vi "G-Unicode Constant Editor.vi"(6 "Variant in":variant, 7 "Shift Pressed?":bool, 8 "error in (no error)":errorcluster, 10 "QD Combo Box Ref":refnum<vi>, 11 "QD Launch VI Ref":refnum<vi>) -> (0 "error out":errorcluster, 4 "Variant out":variant)   [LabVIEW 2020]
doc: "View and edit a constant UTF-8 string or UTF-8 path.\n\nDefault Shortcut - [G]"
uses:
  Types/UTF-8 String/UTF-8 String.lvclass
  Types/UTF-8 String/UTF-8 String.lvclass/UTF-8 String.ctl
  cd947f18-06e6-4942-b232-f387c9ba60e9.vi
  Private/Conversion/String as Encoded String.vi
  Private/Conversion/Polymorphic VIs/String as Encoded String (LabVIEW String).vi
  Private/Conversion/Polymorphic VIs/String as Encoded String (UTF-8 String).vi
  Types/UTF-8 String/Write Encoded UTF-8 String.vi
  Private/Conversion/Text to UTF-8.vi
  Private/Conversion/Polymorphic VIs/Text to UTF-8 (LabVIEW String).vi
  Types/UTF-8 String/Read Encoded UTF-8 String.vi
  Private/Library/gu_input_box.vi
  aec64f6a-b3cd-45af-92d8-e7d8603af3b4.vi
  Types/UTF-8 Path/UTF-8 Path.lvclass
  98fca13f-b951-49ec-b676-3ccf9bd4e781.vi
  5e95c1c1-3841-484b-b44d-c44c65ed04ae.vi
panel:
  in  "Undo Name":string="Quick Drop Keyboard Shortcut"
  # "Do not change the connector pane of this VI.\n\nSee the block diagram for directions on how to use this template."
  # "Specify the name of the Undo transaction"
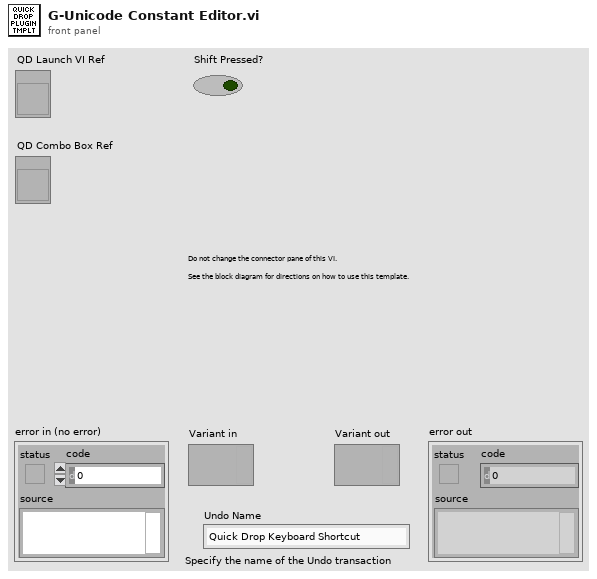
[diagram p1: front panel]
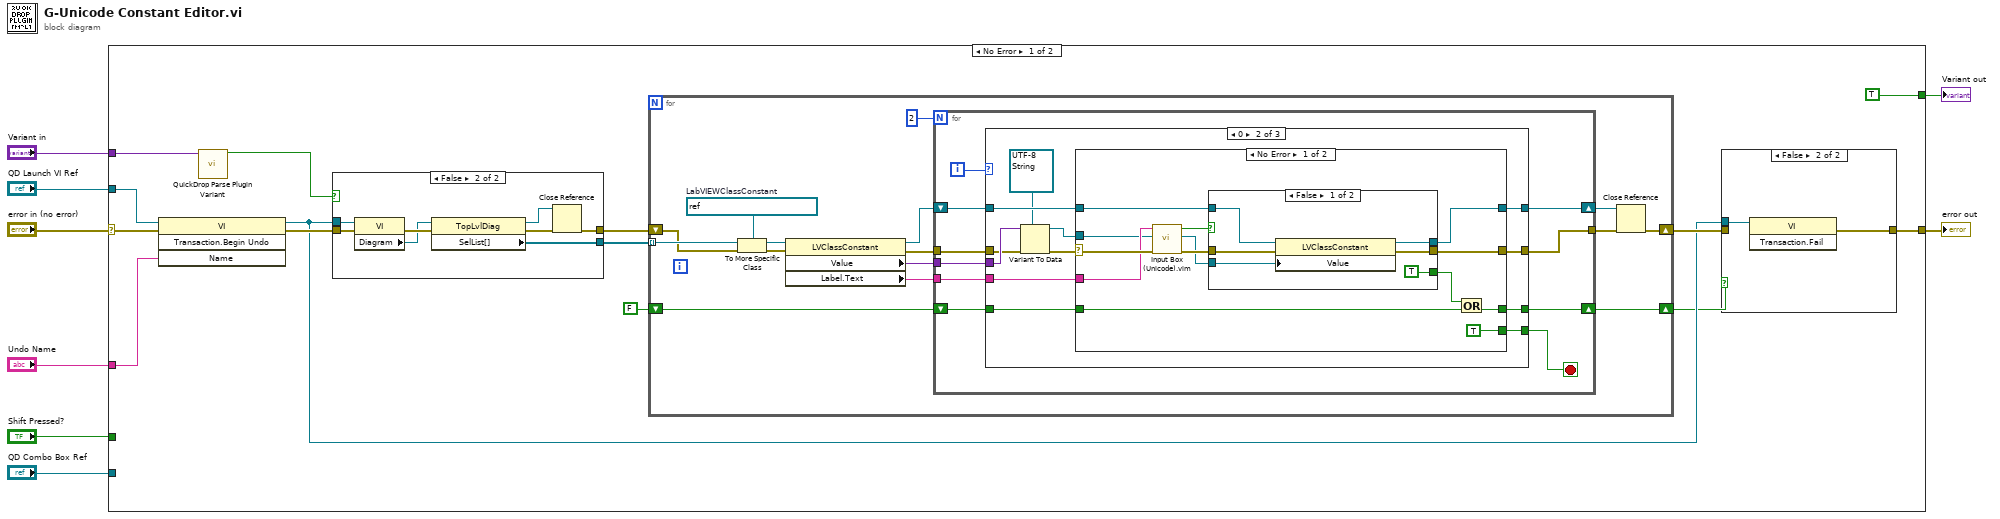
[diagram p0: block diagram]
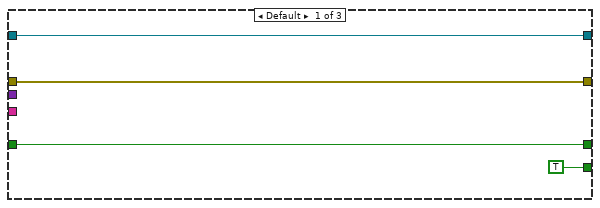
[diagram p2: hidden frame]
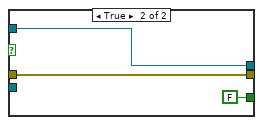
[diagram p3: hidden frame]
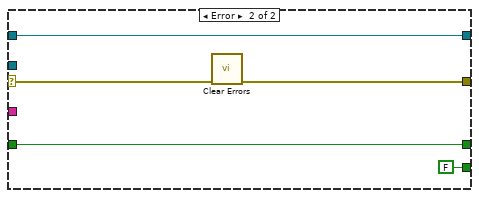
[diagram p4: hidden frame]
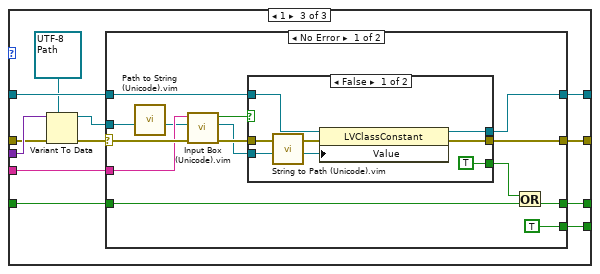
[diagram p5: hidden frame]
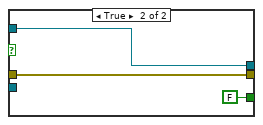
[diagram p6: hidden frame]
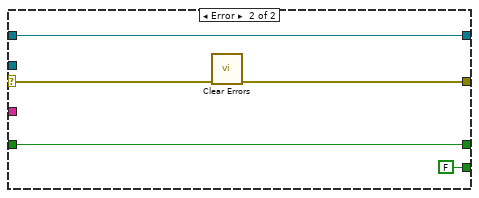
[diagram p7: hidden frame]
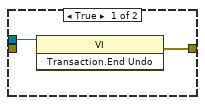
[diagram p8: hidden frame]
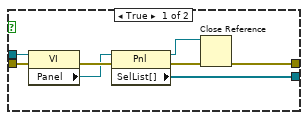
[diagram p9: hidden frame]
diagram:
  n1 = case shown="No Error" "error in (no error)" {
    selector: "error in (no error)" -> [w21 w152]
    tunnel: [w15 w152] -> w7
    tunnel: "QD Launch VI Ref" -> [w20 _]
    tunnel: "Shift Pressed?" -> [_ _]
    tunnel: "QD Combo Box Ref" -> [_ _]
    tunnel: "Variant in" -> [w22 _]
    tunnel: "Undo Name" -> [w19 _]
    tunnel: [TRUE _] -> w1
    frame No Error {
      n2 = invoke class="VI" method="Transaction.Begin Undo"(reference=w20, error in=w21, "Name"=w19) -> (reference out=w12:refnum<vi>, error out=w16:errorcluster)  [unwired: 1 in, 2 out]
      n3 = call <vilib>:"QuickDrop Parse Plugin Variant.vi"("QDKS Variant in"=w22) -> ("QD Launch VI Panel?"=w17:bool)  [unwired: 12 in, 2 out]
      n4 = case shown="False" w17 {
        tunnel: w16 -> [w143 w151]
        tunnel: w12 -> [w142 w150]
        tunnel: [w137 w145] -> w14
        tunnel: [w136 w144] -> w9
        frame True {
          n5 = property class="VI"(reference=w142, error in=w143) -> (error out=w141:errorcluster, "Panel"=w140:refnum<vi>)  [unwired: 1 out]
          n6 = property class="Pnl"(reference=w140, error in=w141) -> (reference out=w138:refnum<vi>, error out=w139:errorcluster, "SelList[]"=w136:refnum<vi>[])
          n7 = Close Reference(reference=w138, error in (no error)=w139) -> (error out=w137:errorcluster)
        }
        frame False {
          n8 = property class="VI"(reference=w150, error in=w151) -> (error out=w149:errorcluster, "Diagram"=w148:refnum<vi>)  [unwired: 1 out]
          n9 = property class="TopLvlDiag"(reference=w148, error in=w149) -> (reference out=w146:refnum<vi>, error out=w147:errorcluster, "SelList[]"=w144:refnum<vi>[])
          n10 = Close Reference(reference=w146, error in (no error)=w147) -> (error out=w145:errorcluster)
        }
      }
      n11 = for {
        shift-right: [w35] -> w13
        shift-left: w14 -> [w31]
        shift-right: [w36] -> w10
        shift-left: FALSE -> [w37]
        tunnel: w9 -> [w34] mode=indexing
        w33 = refnum<vi> refnum  # LabVIEWClassConstant
        n12 = To More Specific Class(target class=w33, reference=w34, error in=w31) -> (specific class reference=w32:refnum<vi>, error out=w30:errorcluster)
        n13 = property class="LVClassConstant"(reference=w32, error in=w30) -> (reference out=w27:refnum<vi>, error out=w28:errorcluster, "Value"=w29:variant, "Label.Text"=w26:string)
        n14 = for {
          N: 2 -> [_]
          tunnel: w29 -> [w45]
          tunnel: w28 -> [w44]
          tunnel: w26 -> [w42]
          tunnel: [w41] -> w25
          shift-right: [w40] -> w24
          shift-left: w27 -> [w43]
          shift-right: [w46] -> w36
          shift-left: w37 -> [w47]
          i -> [w39]
          stop <- w38 stop-if-true
          n15 = case shown="0" w39 {
            tunnel: w47 -> [w50 w63 w102]
            tunnel: [w50 w62 w101] -> w46
            tunnel: w45 -> [_ w61 w100]
            tunnel: w44 -> [w48 w60 w99]
            tunnel: w43 -> [w49 w59 w98]
            tunnel: w42 -> [_ w58 w97]
            tunnel: [w48 w55 w94] -> w41
            tunnel: [w49 w54 w93] -> w40
            tunnel: [TRUE w52 w91] -> w38
            frame Default {
            }
            frame 0 {
              n16 = Variant To Data(error in=w60, type=refnum<class "UTF-8 String.lvclass"> refnum ("G-Unicode.lvlib:UTF-8 String.lvclass"), Variant=w61) -> (data=w56:refnum<class "UTF-8 String.lvclass">, error out=w53:errorcluster)
              n17 = case shown="No Error" w53 {
                selector: w53 -> [w68 w90]
                tunnel: w63 -> [w76 w87]
                tunnel: [w75 w87] -> w62
                tunnel: w56 -> [w65 _]
                tunnel: [w67 w89] -> w55
                tunnel: w59 -> [w70 w88]
                tunnel: [w69 w88] -> w54
                tunnel: w58 -> [w66 _]
                tunnel: [TRUE FALSE] -> w52
                frame No Error {
                  n18 = call "Input Box (Unicode).vim"("error in"=w68, "Default Input"=w65, "Message"=w66) -> ("error out"=w74:errorcluster, "Input"=w72:refnum<class "UTF-8 String.lvclass">, "Cancelled"=w73:bool)  [unwired: 6 in]
                  n19 = case shown="False" w73 {
                    tunnel: w74 -> [w82 w84]
                    tunnel: [w81 w84] -> w67
                    tunnel: w72 -> [w77 _]
                    tunnel: [TRUE ("x") FALSE ("x")] -> w71
                    tunnel: w70 -> [w79 w83]
                    tunnel: [w78 w83] -> w69
                    frame False {
                      n20 = property class="LVClassConstant"(reference=w79, error in=w82, "Value"=w77) -> (reference out=w78:refnum<vi>, error out=w81:errorcluster)
                    }
                    frame True {
                    }
                  }
                  n21 = Or(x=w71, y=w76) -> (x .or. y?=w75:bool)
                }
                frame Error {
                  n22 = call <vilib>:"Clear Errors.vi"("error in (no error)"=w90) -> ("error out"=w89:errorcluster)  [unwired: 5 in, 1 out]
                }
              }
            }
            frame 1 {
              n23 = Variant To Data(error in=w99, type=refnum<class "UTF-8 Path.lvclass"> refnum ("G-Unicode.lvlib:UTF-8 Path.lvclass"), Variant=w100) -> (data=w95:refnum<class "UTF-8 Path.lvclass">, error out=w92:errorcluster)
              n24 = case shown="No Error" w92 {
                selector: w92 -> [w108 w131]
                tunnel: w102 -> [w116 w128]
                tunnel: [w115 w128] -> w101
                tunnel: w95 -> [w105 _]
                tunnel: [w107 w130] -> w94
                tunnel: w98 -> [w110 w129]
                tunnel: [w109 w129] -> w93
                tunnel: w97 -> [w106 _]
                tunnel: [TRUE FALSE] -> w91
                frame No Error {
                  n25 = call "Path to String (Unicode).vim"("Path"=w105) -> ("String"=w103:refnum<class "UTF-8 String.lvclass">)  [unwired: 9 in, 1 out]
                  n26 = call "Input Box (Unicode).vim"("error in"=w108, "Default Input"=w103, "Message"=w106) -> ("error out"=w114:errorcluster, "Input"=w112:refnum<class "UTF-8 String.lvclass">, "Cancelled"=w113:bool)  [unwired: 6 in]
                  n27 = case shown="False" w113 {
                    tunnel: w114 -> [w123 w125]
                    tunnel: [w122 w125] -> w107
                    tunnel: w112 -> [w118 _]
                    tunnel: [TRUE ("x") FALSE ("x")] -> w111
                    tunnel: w110 -> [w120 w124]
                    tunnel: [w119 w124] -> w109
                    frame False {
                      n28 = call "String to Path (Unicode).vim"("String"=w118) -> ("Path"=w117:refnum<class "UTF-8 Path.lvclass">)  [unwired: 9 in, 1 out]
                      n29 = property class="LVClassConstant"(reference=w120, error in=w123, "Value"=w117) -> (reference out=w119:refnum<vi>, error out=w122:errorcluster)
                    }
                    frame True {
                    }
                  }
                  n30 = Or(x=w111, y=w116) -> (x .or. y?=w115:bool)
                }
                frame Error {
                  n31 = call <vilib>:"Clear Errors.vi"("error in (no error)"=w131) -> ("error out"=w130:errorcluster)  [unwired: 5 in, 1 out]
                }
              }
            }
          }
        }
        n32 = Close Reference(reference=w24, error in (no error)=w25) -> (error out=w35:errorcluster)
      }
      n33 = case shown="False" w10 {
        tunnel: w12 -> [w132 w134]
        tunnel: [w133 w135] -> w15
        tunnel: w13 -> [_ _]
        frame True {
          n34 = invoke class="VI" method="Transaction.End Undo"(reference=w132) -> (error out=w133:errorcluster)  [unwired: 2 in, 2 out]
        }
        frame False {
          n35 = invoke class="VI" method="Transaction.Fail"(reference=w134) -> (error out=w135:errorcluster)  [unwired: 2 in, 2 out]
        }
      }
    }
    frame Error {
    }
  }
  "error out" <- w7
  "Variant out" <- w1
